vi "TestInit.vi"(4 "ConfigData":string, 5 "MotorName":string) -> (0 "Parameter OK":bool, 1 "MotorData":T1, 2 "VI Refnum":refnum<vi>)   [LabVIEW 2020]
uses:
  <vilib>/Utility/error.llb/DialogType.ctl
panel:
  out "Keys":string[](array[string])
  out "Input":string[](array[string])
  in  "EPSONC4ID":refnum<k5>
  out "error out":errorcluster
  in  "ID":string
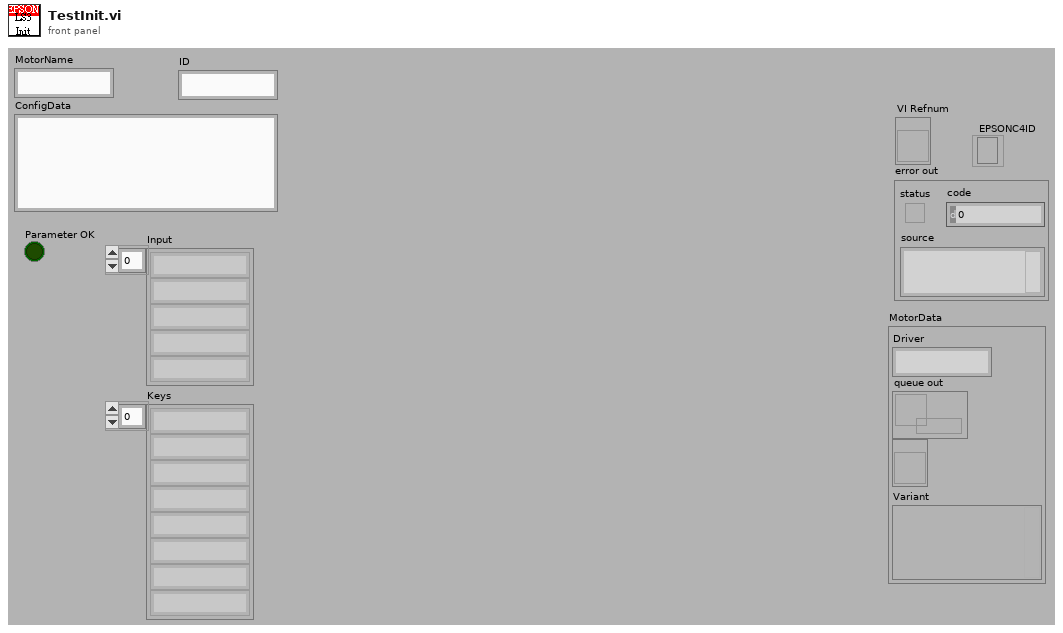
[diagram p1: front panel]
types:
  T1 = cluster{"Driver":string, "queue out":refnum<queue>, refnum<vi>, "Variant":variant}
  T2 = cluster{"Command":string, "Parameter":string, "queue out":refnum<queue>}
  T3 = typedef "DialogType.ctl" = u16
  T4 = cluster{"EPSONC4ID":refnum<k5>, "trimmed string":string, "trimmed string":string}
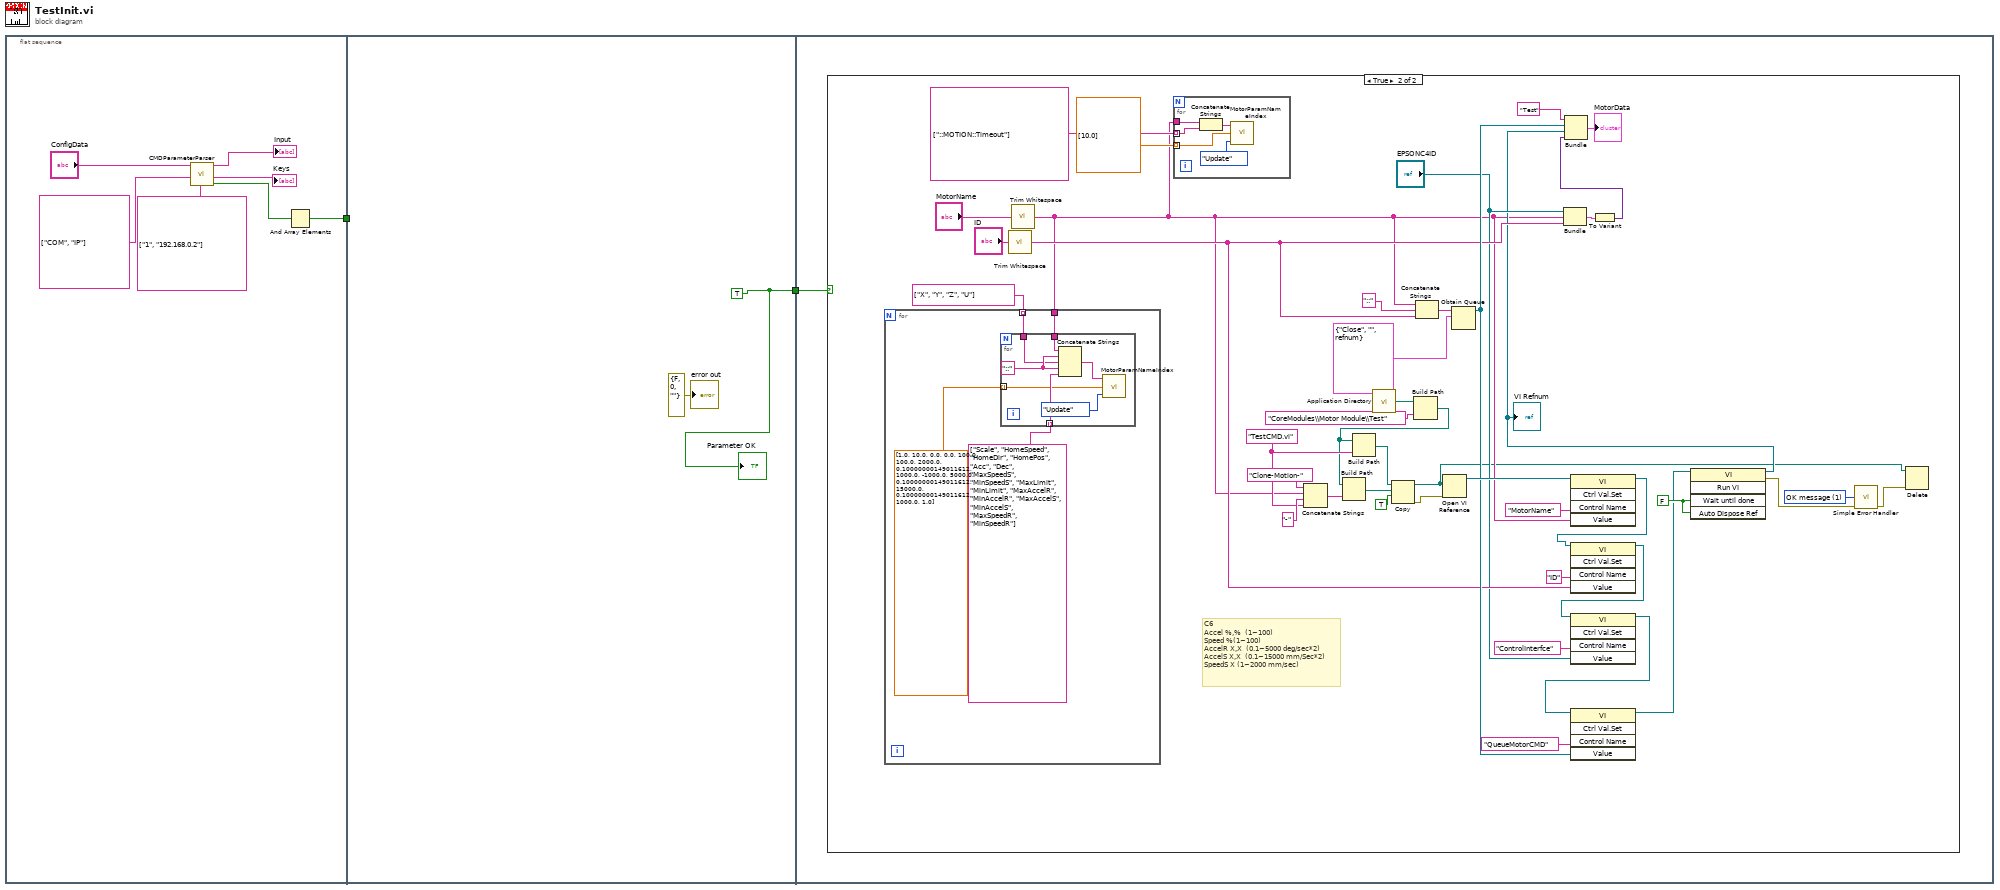
[diagram p0: block diagram]
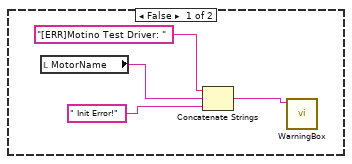
[diagram p2: hidden frame]
diagram:
  n1 = flat-sequence {
    tunnel: [w3] -> w1
    tunnel: [w10] -> w2
    tunnel: w1 -> [_]
    tunnel: w2 -> [w12]
    frame #0 {
      n2 = call "CMDParameterParser.vi"("DeafultValues"=string[] ["1", "192.168.0.2"] ("DeafultValue"), "RequiredKeys"=string[] ["COM", "IP"] ("ParameterKey"), "CMDParameter"="ConfigData") -> ("KeyFind?"=w4:bool[], "KeyValues"=→"Keys":string[], "Input"=→"Input":string[])  [unwired: 6 in]
      n3 = And Array Elements(Boolean array=w4) -> (logical AND=w3:bool)
    }
    frame #1 {
      w10 = TRUE
      "error out" <- errorcluster {"status"=FALSE, "code"=0, "source"=""} ("error out")
      "Parameter OK" <- w10
    }
    frame #2 {
      n4 = case shown="True" w12 {
        frame False {
          n5 = local read "MotorName"() -> (w16:string)
          n6 = Concatenate Strings("[ERR]Motino Test Driver: " ("Mssage"), w16, " Init Error!" ("Mssage")) -> (w13:string)
          n7 = call "WarningBox.vi"("!!!!!!!!!!!!!!!Warning!!!!!!!!!!!!!!"=w13) -> ()  [unwired: 10 in, 1 out]
        }
        frame True {
          w20 = T3 1 items=["no dialog", "OK message", "continue or stop message", "OK message + warnings", "continue/stop + warnings"] ("type of dialog (OK msg:1)")
          w22 = FALSE ("Wait Until Done")
          w49 = "TestCMD.vi" ("name or relative path")
          # "C6\nAccel %,%  (1~100)\nSpeed %(1~100)\nAccelR X,X  (0.1~5000 deg/sec*2)\nAccelS X,X  (0.1~15000 mm/Sec*2)\nSpeedS X (1~2000 mm/sec)"
          n8 = call <vilib>:"Trim Whitespace.vi"("string"="ID") -> ("trimmed string"=w36:string)  [unwired: 1 in]
          n9 = call <vilib>:"Trim Whitespace.vi"("string"="MotorName") -> ("trimmed string"=w24:string)  [unwired: 1 in]
          n10 = for {
            tunnel: w24 -> [w66]
            tunnel: string[] ["X", "Y", "Z", "U"] -> [w64] mode=indexing
            n11 = for {
              tunnel: w66 -> [w71]
              tunnel: w64 -> [w70]
              tunnel: string[] ["Scale", "HomeSpeed", "HomeDir", "HomePos", "Acc", "Dec", "MaxSpeedS", "MinSpeedS", "MaxLimit", "MinLimit", "MaxAccelR", "MinAccelR", "MaxAccelS", "MinAccelS", "MaxSpeedR", "MinSpeedR"] -> [w69] mode=indexing
              tunnel: sgl[] [1.0, 10.0, 0.0, 0.0, 100.0, 100.0, 2000.0, 0.1, 1000.0, -1000.0, 5000.0, 0.1, 15000.0, 0.1, 1000.0, 1.0] -> [w68] mode=indexing
              w74 = "::" ("string")
              n12 = Concatenate Strings(w71, w74, w70, w74, w69) -> (w73:string)
              n13 = call "MotorParamNameIndex.vi"("OP"=enum16{"Get", "Update", "Init"}."Update", "ParamIn"=w68, "ParameterName"=w73) -> ()  [unwired: 3 out]
            }
          }
          n14 = for {
            tunnel: w24 -> [w62]
            tunnel: string[] ["::MOTION::Timeout"] -> [w60] mode=indexing
            tunnel: sgl[] [10.0] -> [w59] mode=indexing
            n15 = Concatenate Strings(w62, w60) -> (w63:string)
            n16 = call "MotorParamNameIndex.vi"("OP"=enum16{"Get", "Update", "Init"}."Update", "ParamIn"=w59, "ParameterName"=w63) -> ()  [unwired: 3 out]
          }
          n17 = Concatenate Strings("Clone-Motion-" ("string"), w24, "-" ("string"), w49) -> (w53:string)
          n18 = call <vilib>:"Application Directory.vi"() -> ("Application Directory"=w29:path)
          n19 = Build Path(base path=w29, name or relative path="CoreModules\\Motor Module\\Test") -> (appended path=w27:path)
          n20 = Build Path(base path=w27, name or relative path=w53) -> (appended path=w51:path)
          n21 = Build Path(base path=w27, name or relative path=w49) -> (appended path=w48:path)
          n22 = Copy(9:TRUE ("overwrite (F)"), 10:w51, 11:w48) -> (0:w23:errorcluster, 3:w18:path)  [unwired: 2 in, 1 out]
          n23 = Concatenate Strings(w24, "::" ("string"), w36) -> (w57:string)
          n24 = Open VI Reference(vi path=w18, error in (no error)=w23) -> (vi reference=w43:refnum<vi>)  [unwired: 4 in, 1 out]
          n25 = Obtain Queue(name (unnamed)=w57, element data type=T2 {"Command"="Close", "Parameter"="", "queue out"=refnum} ("Motor Module CMD")) -> (queue out=w42:refnum<queue>)  [unwired: 3 in, 2 out]
          n26 = Bundle("EPSONC4ID"="EPSONC4ID", "trimmed string"=w24, "trimmed string"=w36) -> (w58:T4)  [unwired: 1 in]
          n27 = invoke class="VI" method="Ctrl Val.Set"(reference=w43, "Control Name"="MotorName", "Value"=w24) -> (reference out=w41:refnum<vi>)  [unwired: 2 in, 4 out]
          n28 = invoke class="VI" method="Ctrl Val.Set"(reference=w41, "Control Name"="ID", "Value"=w36) -> (reference out=w40:refnum<vi>)  [unwired: 2 in, 4 out]
          n29 = invoke class="VI" method="Ctrl Val.Set"(reference=w40, "Control Name"="ControlInterfce", "Value"="EPSONC4ID") -> (reference out=w39:refnum<vi>)  [unwired: 2 in, 4 out]
          n30 = invoke class="VI" method="Ctrl Val.Set"(reference=w39, "Control Name"="QueueMotorCMD", "Value"=w42) -> (reference out=w19:refnum<vi>)  [unwired: 2 in, 4 out]
          n31 = To Variant(anything=w58) -> (Variant=w32:variant)
          n32 = invoke class="VI" method="Run VI"(reference=w19, "Wait until done"=w22, "Auto Dispose Ref"=w22) -> (reference out=w31:refnum<vi>, error out=w21:errorcluster)  [unwired: 2 in, 3 out]
          "VI Refnum" <- w31
          n33 = Bundle("Driver"="Test", "queue out"=w42, w31, "Variant"=w32) -> (→"MotorData":T1)  [unwired: 1 in]
          n34 = call <vilib>:"Simple Error Handler.vi"("type of dialog (OK msg:1)"=w20, "error in (no error)"=w21) -> ("error out"=w17:errorcluster)  [unwired: 3 in, 4 out]
          n35 = Delete(path (use dialog)=w18, error in=w17) -> ()  [unwired: 3 in, 3 out]
        }
      }
    }
  }
